vi "Untitled 2.vi"(6 "PID Config":T1 {"Max I Accu"."Low" format="%#.8f"; "Max I Accu"."High" format="%#.8f"; "Gains"."F" format="%#.8f"; "Gains"."D" format="%#.8f"; "Gains"."I" format="%#.8f"; "Gains"."P" format="%#.8f"; "Error Allowed"."Low" format="%#.8f"; "Error Allowed"."High" format="%#.8f"; "I Zone"."Low" format="%#.8f"; "I Zone"."High" format="%#.8f"; "Max Out"."REV" format="%.2f"; "Max Out"."FWD" format="%.2f"}, 7 "Output":bool, 9 "Auto Target (ft) in":dbl, 10 "PID Enabled Out":bool, 11 "Error Out":dbl) -> (1 "PID Enabled":bool, 2 "Auto error":dbl, 3 "Boolean":bool, 4 "Auto Target (ft) out":dbl)   [LabVIEW 2023, in "Thor-SwerveDrive_ACT.lvlib"]
uses:
  Thor-SwerveDrive_ACT.lvlib
  Shared Code/TypeDefs/Cluster_FWD  REV Values.ctl
  Shared Code/TypeDefs/Cluster_High-Low.ctl
  Shared Code/TypeDefs/Cluster_PID Gains.ctl
  Shared Code/TypeDefs/Cluster_PID Config.ctl
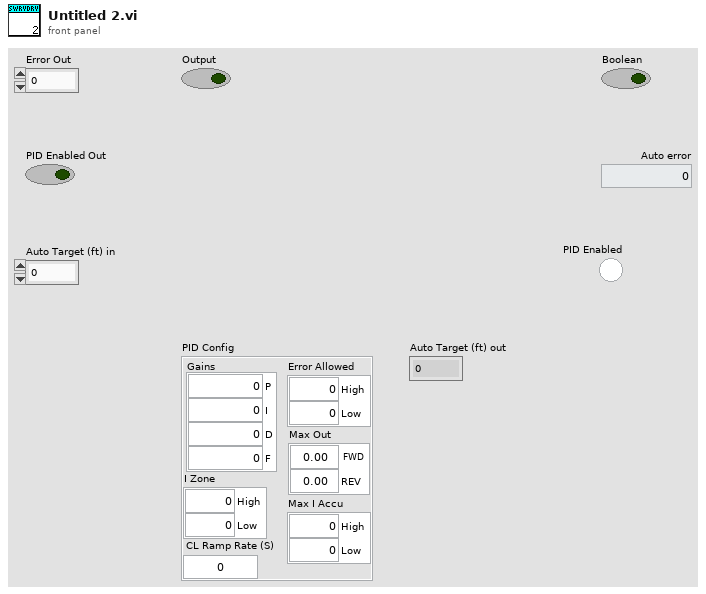
[diagram p1: front panel]
types:
  T1 = typedef "Cluster_PID Config.ctl" = cluster{"Gains":T2, "Error Allowed":T3, "I Zone":T3, "Max Out":T4, "Max I Accu":T3, "CL Ramp Rate (S)":dbl}
  T2 = typedef "Cluster_PID Gains.ctl" = cluster{"P":dbl, "I":dbl, "D":dbl, "F":dbl}
  T3 = typedef "Cluster_High-Low.ctl" = cluster{"High":dbl, "Low":dbl}
  T4 = typedef "Cluster_FWD  REV Values.ctl" = cluster{"FWD":dbl, "REV":dbl}
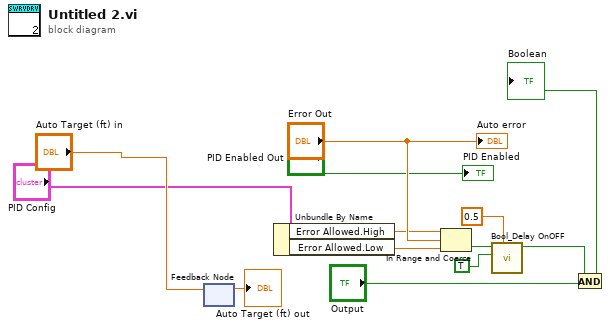
[diagram p0: block diagram]
diagram:
  n1 = feedback #1() -> (→"Auto Target (ft) out":dbl)  [unwired: 1 in]
  n2 = feedback-in #1("Auto Target (ft) in") -> ()
  n3 = Unbundle By Name("PID Config") -> ("Error Allowed.High"=w3:dbl, "Error Allowed.Low"=w4:dbl)
  n4 = In Range and Coerce(upper limit=w3, x="Error Out", lower limit=w4) -> (In Range?=w9:bool)  [unwired: 1 out]
  n5 = call "Bool_Delay OnOFF.vi"("Delay Time(S)"=0.5, "Delay On(t) Off(f)"=TRUE, "Input"=w9) -> ("Output"=w12:bool)  [unwired: 7 in, 1 out]
  n6 = And(x=w12, y="Output") -> (x .and. y?=→"Boolean":bool)
  "Auto error" <- "Error Out"
  "PID Enabled" <- "PID Enabled Out"
